vi "PID No Jump.vi"(4 "Initial output":dbl format="%.2f", 5 "swing":dbl format="%.2f", 6 "reinitialize? (F)":bool, 7 "output range":cluster{"output high":dbl, "output low":dbl}={"output high"=100.0, "output low"=-100.0} {"output low" format="%.2f"; "output high" format="%.2f"}, 9 "PID gains":T1={"proportional gain (Kc)"=1.0, "integral time (Ti, min)"=0.01, "derivative time (Td, min)"=0.0} {"derivative time (Td, min)" format="%.3f"; "integral time (Ti, min)" format="%.3f"; "proportional gain (Kc)" format="%.3f"}, 10 "process variable":dbl format="%.2f", 11 "setpoint":dbl format="%.2f") -> (3 "output":dbl)   [LabVIEW 2013]
uses:
  <vilib>/addons/control/pid/pid.llb/PID (DBL).vi
  <vilib>/addons/control/pid/NI_PID_pid.lvlib
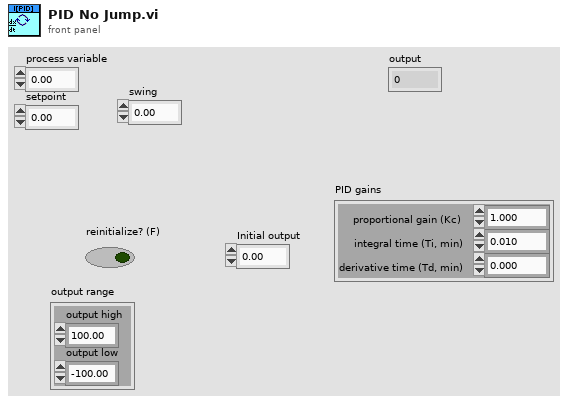
[diagram p1: front panel]
types:
  T1 = cluster{"proportional gain (Kc)":dbl, "integral time (Ti, min)":dbl, "derivative time (Td, min)":dbl}
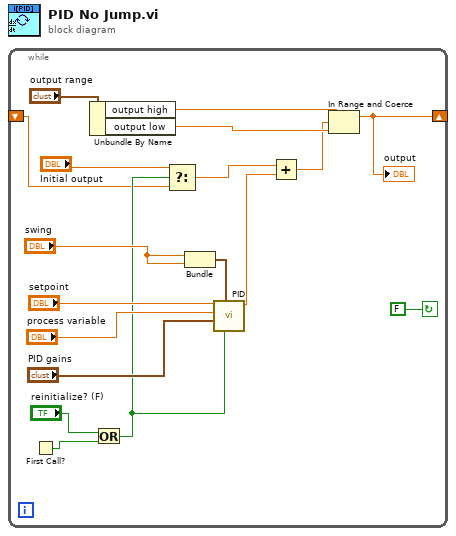
[diagram p0: block diagram]
diagram:
  n1 = while {
    shift-right: [w9] -> _
    shift-left: _ -> [w2]
    stop <- FALSE continue-if-true
    n2 = First Call?() -> (First Call?: T/F=w5:bool)
    n3 = Unbundle By Name("output range") -> ("output high"=w12:dbl, "output low"=w11:dbl)
    n4 = Or(x="reinitialize? (F)", y=w5) -> (x .or. y?=w4:bool)
    n5 = Select(t="Initial output", s=w4, f=w2) -> (s? t:f=w1:dbl)
    n6 = Bundle("swing"="swing", "swing"="swing") -> (w8:cluster{"swing":dbl, "swing":dbl})  [unwired: 1 in]
    n7 = call-poly <vilib>:"PID.vi"("reinitialize? (F)"=w4, "output range"=w8, "PID gains"="PID gains", "process variable"="process variable", "setpoint"="setpoint") -> ("output"=w17:dbl)  [unwired: 5 in, 1 out]
    n8 = Add(x=w1, y=w17) -> (x+y=w10:dbl)
    n9 = In Range and Coerce(upper limit=w12, x=w10, lower limit=w11) -> (coerced(x)=w9:dbl)  [unwired: 1 out]
    "output" <- w9
  }
